vi "工具_获取未激活的应用序号.vi"(8 "error in (no error)":errorcluster caption="错误输入（无错误）", 11 "应用信息":T1(array[cluster])) -> (0 "error out":errorcluster caption="错误输出", 3 "未激活应用顺序":i32[](array[numeric]))   [LabVIEW 2014]
doc: "该模板用于创建子VI。"
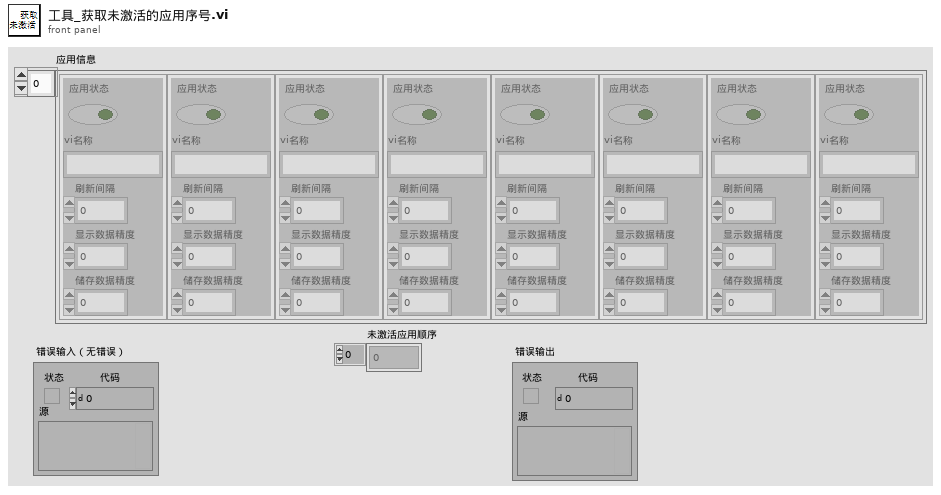
[diagram p1: front panel]
types:
  T1 = cluster{"应用状态":bool, "vi名称":string, "刷新间隔":u32, "显示数据精度":u32, "储存数据精度":u32}[]
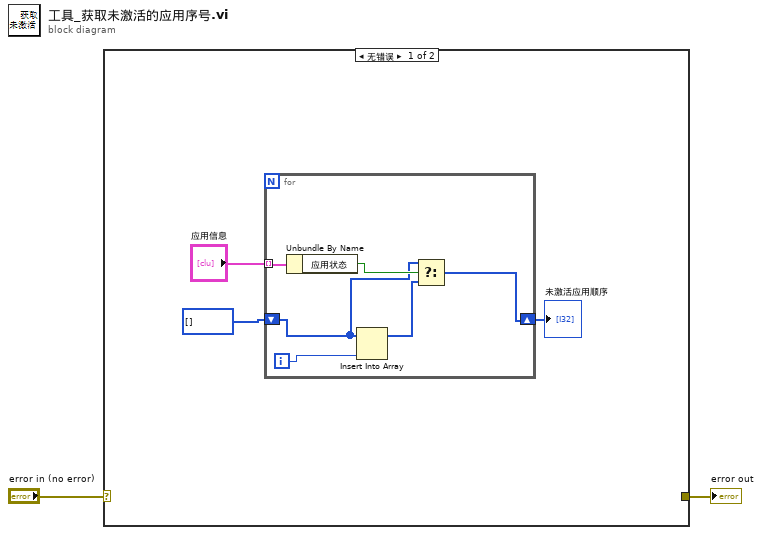
[diagram p0: block diagram]
diagram:
  n1 = case shown="无错误" "error in (no error)" {
    selector: "error in (no error)" -> [_ w12]
    tunnel: [_ w12] -> w1
    frame No Error {
      n2 = for {
        tunnel: "应用信息" -> [w11] mode=indexing
        shift-right: [w6] -> w3
        shift-left: i32[] [] -> [w8]
        i -> [w9]
        n3 = Unbundle By Name(w11) -> ("应用状态"=w10:bool)
        n4 = Insert Into Array(array=w8, new element=w9) -> (w7:i32[])  [unwired: 1 in]
        n5 = Select(t=w8, s=w10, f=w7) -> (s? t:f=w6:i32[])
      }
      "未激活应用顺序" <- w3
    }
    frame Error {
    }
  }
  "error out" <- w1
